vi "HindbrainLIDAR_Sim.vi"(11 "SubPosition":cluster{"xsub":dbl, "ysub":dbl, "heading":dbl}) -> (3 "WhatAroundMe?":cluster{"T":dbl, "Range":dbl, "Bearing":dbl}[](array[cluster]))   [LabVIEW 2012]
doc: "The SimLIDAR subVI takes test track image reference data and the intitailized LIDAR data from the Forebrain VI and injects it into the \"What is Around me?\" data flow at the FPGA level in the Hindbrain.\n\nInput cluster x\n y\n heading\nOutput cluster T\n Range\n Bearing"
panel:
  # "This SubVI simulates the LIDAR data\nthe robot would see on any given\nMap.jpg test track"
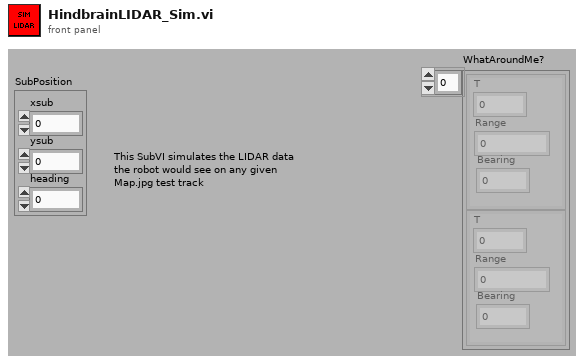
[diagram p1: front panel]
types:
  T1 = cluster{"NumberOfBeams":i32, "SonarRange":dbl, "Noise (0.1 to 1)":dbl}
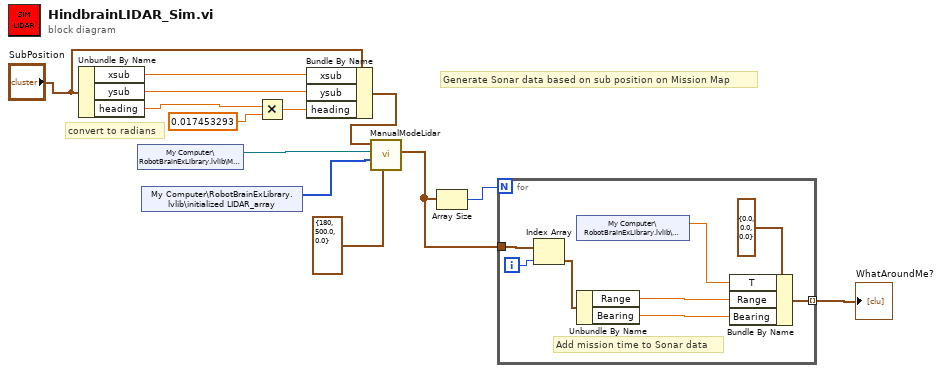
[diagram p0: block diagram]
diagram:
  # "convert to radians"
  # "Generate Sonar data based on sub position on Mission Map"
  n1 = Unbundle By Name("SubPosition") -> ("xsub"=w4:dbl, "ysub"=w5:dbl, "heading"=w3:dbl)
  n2 = shared-variable "My Computer\\RobotBrainExLibrary.lvlib\\MDF Image"() -> (w11:refnum<image>)  [unwired: 1 in, 1 out]
  n3 = shared-variable "My Computer\\RobotBrainExLibrary.lvlib\\initialized LIDAR_array"() -> (w12:i32[])  [unwired: 1 in, 1 out]
  n4 = Multiply(x=w3, y=0.017453293) -> (x*y=w2:dbl)
  n5 = Bundle By Name(cluster="SubPosition", "xsub"=w4, "ysub"=w5, "heading"=w2) -> (w6:cluster{"xsub":dbl, "ysub":dbl, "heading":dbl})
  n6 = call "ManualModeLidar.vi"("LIDARControl"=T1 {"NumberOfBeams"=180, "SonarRange"=500.0, "Noise (0.1 to 1)"=0.0}, "initialized \nsonar ray\narray"=w12, "MDF Image"=w11, "SubPosition"=w6) -> ("LIDAR Data (r:pixel b:degrees)"=w9:cluster{"Range":dbl, "Bearing":dbl}[])  [unwired: 2 in, 3 out]
  n7 = Array Size(array=w9) -> (size(s)=w10:i32)
  n8 = for {
    N: w10 -> [_]
    tunnel: w9 -> [w21]
    tunnel: [w17] -> w8 mode=indexing
    i -> [w20]
    # "Add mission time to Sonar data"
    n9 = Index Array "Index Array"(array=w21, index=w20) -> (element=w19:cluster{"Range":dbl, "Bearing":dbl})
    n10 = shared-variable "My Computer\\RobotBrainExLibrary.lvlib\\MissionTime"() -> (w16:dbl)  [unwired: 1 in, 1 out]
    n11 = Unbundle By Name "Unbundle By Name"(w19) -> ("Range"=w15:dbl, "Bearing"=w14:dbl)
    n12 = Bundle By Name(cluster=cluster{"T":dbl, "Range":dbl, "Bearing":dbl} {"T"=0.0, "Range"=0.0, "Bearing"=0.0} ("Cluster"), "T"=w16, "Range"=w15, "Bearing"=w14) -> (w17:cluster{"T":dbl, "Range":dbl, "Bearing":dbl})
  }
  "WhatAroundMe?" <- w8
